vi "Create JSON Config String.vi"(3 "JSON Config":string) -> (5 "Config string":string)   [LabVIEW 2021, in "CIFLogs.lvlib"]
uses:
  CIFLogs.lvlib
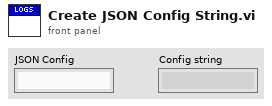
[diagram p1: front panel]
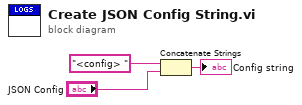
[diagram p0: block diagram]
diagram:
  n1 = Concatenate Strings("<config> ", "JSON Config") -> (→"Config string":string)
